vi "StringCnvPrecision.vi"(0 "Number":dbl, 1 "Header":T1) -> (5 "Float String":string)   [LabVIEW 2018]
uses:
  Controls/HeaderNames.ctl
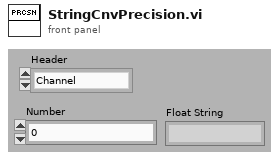
[diagram p1: front panel]
types:
  T1 = typedef "HeaderNames.ctl" = enum16{"Channel", "Device", "Spacer", "Description", "MB", "Range", "Terminal", "Coupling", "Thresh (V)", "Pulse/Rev", "Slope", "Min EU", "Min RPM", "mV/EU", "Iex", "Temp Units", "Type", "CJC Src", "CJC Val", "Ro", "Wire Cfg", "Strain Mode", "Vex", "Bridge Type", "GF", "Gauge Res", "Poisson", "Lead Res", "Init Strain", "GAF", "Scale", "Offset", "Unit (EU)", "dB?", "dB Ref", "Cal Mag", "Cal Units", "Max Temp", "Min Temp", "Max Strain", "Min Strain"}
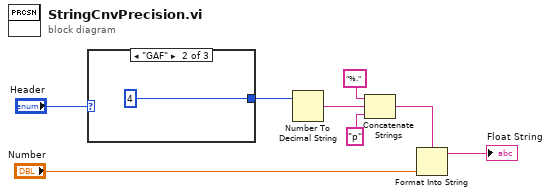
[diagram p0: block diagram]
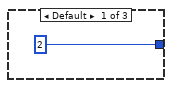
[diagram p2: hidden frame]
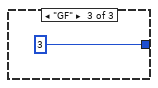
[diagram p3: hidden frame]
diagram:
  n1 = case shown="\"GAF\"" "Header" {
    tunnel: [i16 2 ("precision (6)") i16 4 ("precision (6)") i16 3 ("precision (6)")] -> w6
    frame Default {
    }
    frame "GAF" {
    }
    frame "GF" {
    }
  }
  n2 = Number To Decimal String(number=w6) -> (decimal integer string=w4:string)  [unwired: 1 in]
  n3 = Concatenate Strings("%.", w4, "p" ("string")) -> (w2:string)
  n4 = Format Into String(format string=w2, "Number") -> (resulting string=→"Float String":string)  [unwired: 2 in, 1 out]
